vi "Parameter Set Read.vi"   [LabVIEW 2023, in "Cycler.lvclass"]
uses:
  Cycler.lvclass
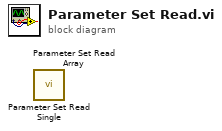
[diagram p0: block diagram]
diagram:
  n1 = call "Parameter Set Read Single.vi"() -> ()  [unwired: 8 in, 4 out]
  n2 = call "Parameter Set Read Array.vi"() -> ()  [unwired: 8 in, 4 out]
